vi "TCP-Send Command.vi"(0 "PXI Address":string, 5 "Port":i32, 7 "Command":string, 9 "timeout (ms)":i32=5000, 11 "error in (no error)":errorcluster, 12 "fast response":bool) -> (15 "error out":errorcluster)   [LabVIEW 2020]
panel:
  out "result":i32
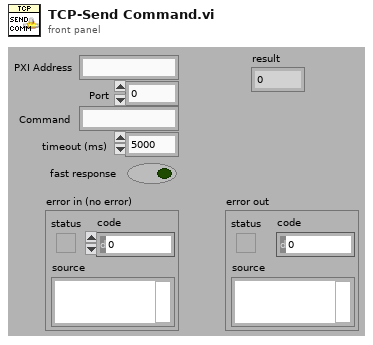
[diagram p1: front panel]
types:
  T1 = enum16{"Standard", "Buffered", "CRLF", "Immediate"}
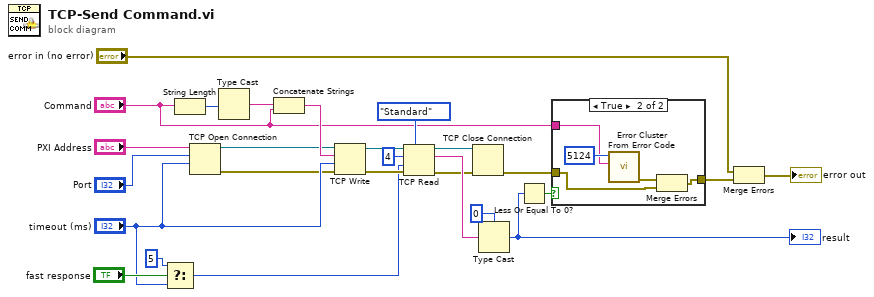
[diagram p0: block diagram]
diagram:
  n1 = Select(t=5 ("timeout ms (25000)"), s="fast response", f="timeout (ms)") -> (s? t:f=w5:i32)
  n2 = String Length(string="Command") -> (length=w23:i32)
  n3 = TCP Open Connection(address="PXI Address", remote port or service name="Port", timeout ms (60000)="timeout (ms)") -> (connection ID=w21:refnum<k5>, error out=w1:errorcluster)  [unwired: 2 in]
  n4 = Type Cast(x=w23) -> (*(type *) &x=w22:string)  [unwired: 1 in]
  n5 = Concatenate Strings(w22, "Command") -> (w24:string)
  n6 = TCP Write(connection ID=w21, data in=w24, error in (no error)=w1, 9:"timeout (ms)") -> (connection ID out=w20:refnum<k5>, error out=w9:errorcluster)  [unwired: 1 out]
  n7 = TCP Read(connection ID=w20, bytes to read=4, error in (no error)=w9, 7:T1."Standard" ("mode (standard)"), 9:w5) -> (connection ID out=w19:refnum<k5>, data out=w18:string, error out=w8:errorcluster)
  n8 = TCP Close Connection(connection ID=w19, error in (no error)=w8) -> (error out=w11:errorcluster)  [unwired: 1 in, 1 out]
  n9 = Type Cast(type=0, x=w18) -> (*(type *) &x=w3:i32)
  "result" <- w3
  n10 = Less Or Equal To 0?(x=w3) -> (x <= 0?=w16:bool)
  n11 = case shown="True" w16 {
    tunnel: [w27 w29] -> w15
    tunnel: w11 -> [w27 w28]
    tunnel: "Command" -> [_ w30]
    frame False {
    }
    frame True {
      n12 = call <vilib>:"Error Cluster From Error Code.vi"("error message (\"\")"=w30, "error code (0)"=5124) -> ("error out"=w32:errorcluster)  [unwired: 7 in]
      n13 = Merge Errors(w32, w28) -> (w29:errorcluster)
    }
  }
  n14 = Merge Errors("error in (no error)", w15) -> (→"error out":errorcluster)
